vi "Update Fields Table for Spartan 5.0.vi"(8 "error in (no error)":errorcluster, 10 "spartan install dir":path, 11 "Connection Refnum":T1) -> (0 "error out":errorcluster, 2 "Map IndexName to FieldId":T2(array[cluster]), 3 "dup Connection Refnum":T1)   [LabVIEW 2011]
uses:
  SI.LIB/ODBC/SQL Controls/Connection Refnum.ctl
  Field Order By.ctl
  Field DataTypes.ctl
  Field Record.ctl
  Field NextItem.ctl
panel:
  out "array":string[](array[string])
  out "Array":errorcluster[](array[cluster])
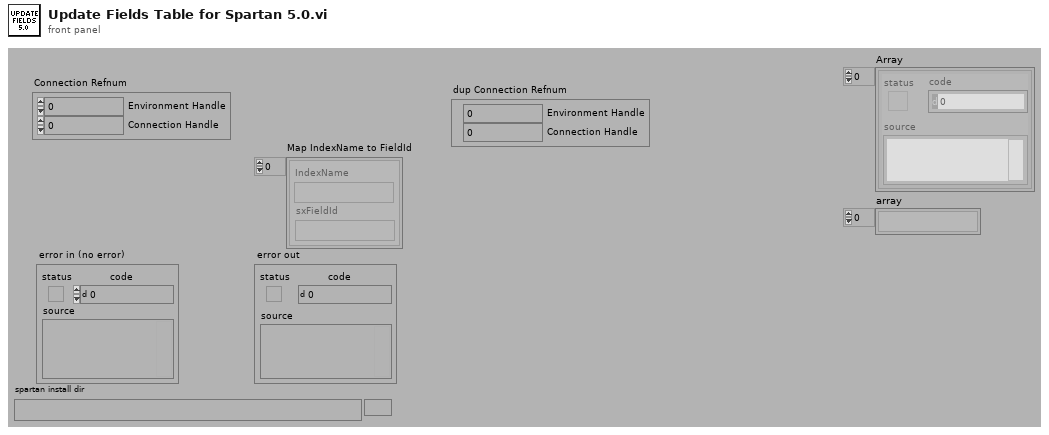
[diagram p1: front panel]
types:
  T1 = typedef "Connection Refnum.ctl" = cluster{"Environment Handle":i32, "Connection Handle":i32}
  T2 = cluster{"IndexName":string, "sxFieldId":string}[]
  T3 = typedef "Field Record.ctl" = cluster{"ixField":i32, "iSequenceOrder":i32, "sxFieldId":string, "sxSequenceId":string, "sDisplayName":string, "sValue":string, "sUnits":string, "nDataType":T4, "nNextItem":T5, "fSystem":bool, "fSystemValue":bool, "fRequired":bool, "fSetAtTest":bool, "fTestField":bool, "fDeleted":bool, "fIndexed":bool, "fFreeList":bool}
  T4 = typedef "Field DataTypes.ctl" = enum32{"text", "numeric", "list", "timestamp", "boolean"}
  T5 = typedef "Field NextItem.ctl" = enum32{"Reset", "Retain", "Auto-Increment"}
  T6 = enum16{"tdm_file", "tdm_channelgroup", "tdm_channel"}
  T7 = typedef "Field Order By.ctl" = enum32{"sxSequenceId", "sxFieldId", "sDisplayName", "sValue", "fSetAtTest", "fRequired", "nNextItem"}
  T8 = typedef "Statement Refnum.ctl" = cluster{"Statement Handle":i32, "Parameter Number":u16}
  T9 = typedef "DataFinder Indexed Property DataTypes.ctl" = enum32{"not optimized", "string", "double", "integer"}
  T10 = cluster{"DisplayName":string, "DataType":T9, "BuiltIn":bool}[]
  T11 = cluster{"DisplayName":string, "sxFieldId":string}
  T12 = cluster{"DisplayName":string, "sxFieldId":string}[]
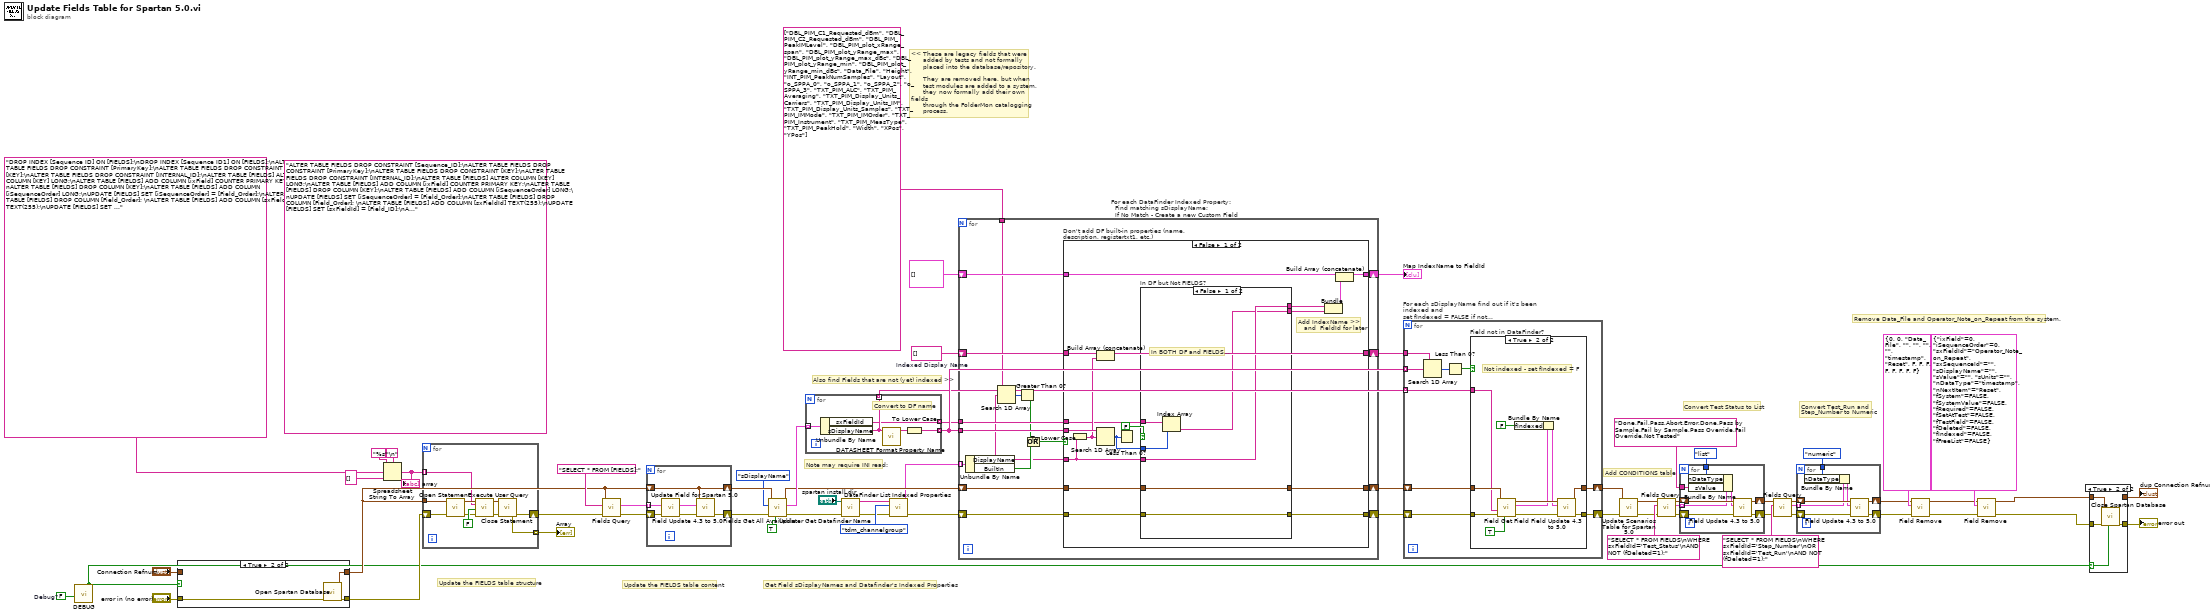
[diagram p0: block diagram]
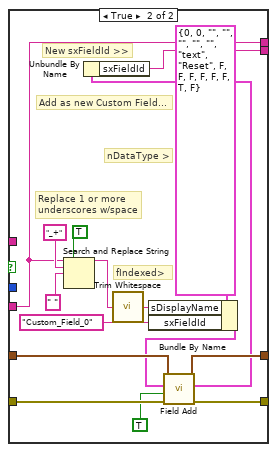
[diagram p5: hidden frame]
diagram:
  w7 = FALSE  # Debug?
  (unwired) "ALTER TABLE FIELDS DROP CONSTRAINT [Sequence_ID];\nALTER TABLE FIELDS DROP CONSTRAINT [PrimaryKey];\nALTER TABLE FIELDS DROP CONSTRAINT [KEY];\nALTER TABLE FIELDS DROP CONSTRAINT [INTERNAL_ID];\nALTER TABLE [FIELDS] ALTER COLUMN [KEY] LONG;\nALTER TABLE [FIELDS] ADD COLUMN [ixField] COUNTER PRIMARY KEY;\nALTER TABLE [FIELDS] DROP COLUMN [KEY];\nALTER TABLE [FIELDS] ADD COLUMN [iSequenceOrder] LONG;\nUPDATE [FIELDS] SET [iSequenceOrder] = [Field_Order];\nALTER TABLE [FIELDS] DROP COLUMN [Field_Order]; \nALTER TABLE [FIELDS] ADD COLUMN [sxFieldId] TEXT(255);\nUPDATE [FIELDS] SET [sxFieldId] = [Field_ID];\nALTER TABLE [FIELDS] DROP COLUMN [Field_ID]; \nALTER TABLE [FIELDS] ADD COLUMN [sxSequenceId] TEXT(255);\nUPDATE [FIELDS] SET [sxSequenceId] = [Sequence_ID] WHERE Sequence_ID IS NOT NULL;\nALTER TABLE [FIELDS] ADD COLUMN [sDisplayName] TEXT(255);\nUPDATE [FIELDS] SET [sDisplayName] = [Display_Name];\nALTER TABLE [FIELDS] DROP COLUMN [Display_Name]; \nALTER TABLE [FIELDS] ADD COLUMN [sValue] TEXT(255);\nUPDATE [FIELDS] SET [sValue] = [Field_Value];\nALTER TABLE [FIELDS] DROP COLUMN [Field_Value];\nALTER TABLE [FIELDS] ADD COLUMN [sUnits] TEXT(255);\nALTER TABLE [FIELDS] ADD COLUMN [nDataType] LONG;\nALTER TABLE [FIELDS] ADD COLUMN [nNextItem] LONG;\nALTER TABLE [FIELDS] ADD COLUMN [fSystem] LONG;\nALTER TABLE [FIELDS] ADD COLUMN [fSystemValue] LONG;\nALTER TABLE [FIELDS] ADD COLUMN [fRequired] LONG;\nALTER TABLE [FIELDS] ADD COLUMN [fSetAtTest] LONG;\nALTER TABLE [FIELDS] ADD COLUMN [fTestField] LONG;\nALTER TABLE [FIELDS] ADD COLUMN [fDeleted] LONG;\nALTER TABLE [FIELDS] ADD COLUMN [fIndexed] LONG;\nALTER TABLE [FIELDS] ADD COLUMN [fFreeList] LONG;\nUPDATE [FIELDS] SET [sUnits] = [Properties];\nALTER TABLE [FIELDS] DROP COLUMN [Properties];\nALTER TABLE [FIELDS] DROP CONSTRAINT [SEQUENCESFIELDS];\nALTER TABLE [FIELDS] DROP COLUMN [Sequence_ID];" ("User Query")
  w53 = string[] []  # Indexed Display Name
  # "<< These are legacy fields that were\n      added by tests and not formally\n      placed into the database/repository.\n\n      They are removed here, but when\n      test modules are added to a system,\n      they now formally add their own fields\n      through the FolderMon catalogging\n      process."
  # "Note may require INI read:"
  # "Convert Test_Run and\nStep_Number to Numeric"
  # "Remove Data_File and Operator_Note_on_Repeat from the system."
  # "Convert Test Status to List"
  # "Also find Fields that are not (yet) indexed >>"
  # "Get Field sDisplayNames and Datafinder's Indexed Properties"
  # "Add CONDITIONS table"
  # "Update the FIELDS table content"
  # "Update the FIELDS table structure"
  n1 = call "DEBUG.vi"("Dev DEBUG? (f)"=w7) -> ("DEBUG?"=w6:bool)  [unwired: 1 in, 5 out]
  n2 = case shown="True" w6 {
    tunnel: "Connection Refnum" -> [w68 _]
    tunnel: "error in (no error)" -> [w67 w71]
    tunnel: [w67 w70] -> w11
    tunnel: [w68 w69] -> w13
    frame False {
    }
    frame True {
      n3 = call "Open Spartan Database.vi"("error in (no error)"=w71) -> ("error out"=w70:errorcluster, "Connection Refnum"=w69:T1)  [unwired: 2 in, 7 out]
    }
  }
  n4 = Spreadsheet String To Array(delimiter (Tab)="\n", format string="%s", spreadsheet string="DROP INDEX [Sequence ID] ON [FIELDS];\nDROP INDEX [Sequence ID1] ON [FIELDS];\nALTER TABLE FIELDS DROP CONSTRAINT [PrimaryKey];\nALTER TABLE FIELDS DROP CONSTRAINT [KEY];\nALTER TABLE FIELDS DROP CONSTRAINT [INTERNAL_ID];\nALTER TABLE [FIELDS] ALTER COLUMN [KEY] LONG;\nALTER TABLE [FIELDS] ADD COLUMN [ixField] COUNTER PRIMARY KEY;\nALTER TABLE [FIELDS] DROP COLUMN [KEY];\nALTER TABLE [FIELDS] ADD COLUMN [iSequenceOrder] LONG;\nUPDATE [FIELDS] SET [iSequenceOrder] = [Field_Order];\nALTER TABLE [FIELDS] DROP COLUMN [Field_Order]; \nALTER TABLE [FIELDS] ADD COLUMN [sxFieldId] TEXT(255);\nUPDATE [FIELDS] SET [sxFieldId] = [Field_ID];\nALTER TABLE [FIELDS] DROP COLUMN [Field_ID]; \nALTER TABLE [FIELDS] ADD COLUMN [sxSequenceId] TEXT(255);\nUPDATE [FIELDS] SET [sxSequenceId] = [Sequence_ID] WHERE Sequence_ID IS NOT NULL;\nALTER TABLE [FIELDS] ADD COLUMN [sDisplayName] TEXT(255);\nUPDATE [FIELDS] SET [sDisplayName] = [Display_Name];\nALTER TABLE [FIELDS] DROP COLUMN [Display_Name]; \nALTER TABLE [FIELDS] ADD COLUMN [sValue] TEXT(255);\nUPDATE [FIELDS] SET [sValue] = [Field_Value];\nALTER TABLE [FIELDS] DROP COLUMN [Field_Value];\nALTER TABLE [FIELDS] ADD COLUMN [sUnits] TEXT(255);\nALTER TABLE [FIELDS] ADD COLUMN [nDataType] LONG;\nALTER TABLE [FIELDS] ADD COLUMN [nNextItem] LONG;\nALTER TABLE [FIELDS] ADD COLUMN [fSystem] LONG;\nALTER TABLE [FIELDS] ADD COLUMN [fSystemValue] LONG;\nALTER TABLE [FIELDS] ADD COLUMN [fRequired] LONG;\nALTER TABLE [FIELDS] ADD COLUMN [fSetAtTest] LONG;\nALTER TABLE [FIELDS] ADD COLUMN [fTestField] LONG;\nALTER TABLE [FIELDS] ADD COLUMN [fDeleted] LONG;\nALTER TABLE [FIELDS] ADD COLUMN [fIndexed] LONG;\nALTER TABLE [FIELDS] ADD COLUMN [fFreeList] LONG;\nUPDATE [FIELDS] SET [sUnits] = [Properties];\nALTER TABLE [FIELDS] DROP COLUMN [Properties];\nALTER TABLE [FIELDS] DROP CONSTRAINT [SEQUENCESFIELDS];\nALTER TABLE [FIELDS] DROP COLUMN [Sequence_ID];" ("User Query"), array type (2D Dbl)=string[] []) -> (array=w65:string[])
  "array" <- w65
  n5 = for {
    tunnel: w13 -> [w77]
    tunnel: w65 -> [w73] mode=indexing
    tunnel: [w72] -> w5 mode=indexing
    shift-right: [w72] -> w33
    shift-left: w11 -> [w74]
    n6 = call "Open Statement.vi"("error in (no error)"=w74, "Connection Refnum"=w77) -> ("error out"=w79:errorcluster, "Statement Refnum"=w78:T8)  [unwired: 4 out]
    n7 = call "Execute User Query.vi"("error in (no error)"=w79, "Return Data? (f)"=FALSE, "User Query"=w73, "Statement Refnum"=w78) -> ("error out"=w75:errorcluster, "Statement Refnum"=w76:T8)  [unwired: 2 out]
    n8 = call "Close Statement.vi"("error in (no error)"=w75, "Statement Refnum"=w76) -> ("error out"=w72:errorcluster)  [unwired: 5 out]
  }
  "Array" <- w5
  n9 = call "Fields Query.vi"("error in (no error)"=w33, "Query"="SELECT * FROM [FIELDS];", "Connection Refnum"=w13) -> ("error out"=w61:errorcluster, "Fields"=w60:T3[])  [unwired: 1 in, 6 out]
  n10 = for {
    shift-right: [w86] -> w32
    shift-left: w61 -> [w83]
    shift-right: [w85] -> w59
    shift-left: w13 -> [w85]
    tunnel: w60 -> [w84] mode=indexing
    n11 = call "Update Field for Spartan 5.0.vi"("error in (no error)"=w83, "Old Field Record"=w84) -> ("error out"=w82:errorcluster, "New Field Record"=w81:T3)  [unwired: 8 out]
    n12 = call "Field Update 4.3 to 5.0.vi"("error in (no error)"=w82, "Field Record"=w81, "Connection Refnum"=w85) -> ("error out"=w86:errorcluster)  [unwired: 8 out]
  }
  n13 = call "Fields Get All Available.vi"("Combine All? (f)"=TRUE, "error in (no error)"=w32, "Sort by (sxSequenceId)"=Field_Order_By."sDisplayName", "Connection Refnum"=w59) -> ("error out"=w28:errorcluster, "System or ALL Combined Fields"=w55:T3[], "Connection Refnum"=w54:T1)  [unwired: 1 in, 4 out]
  n14 = for {
    tunnel: w55 -> [w91] mode=indexing
    tunnel: [w89] -> w49 mode=indexing
    tunnel: [w88] -> w48 mode=indexing
    tunnel: [w87] -> w46 mode=indexing
    # "Convert to DF name"
    n15 = Unbundle By Name(w91) -> ("sxFieldId"=w87:string, "sDisplayName"=w88:string)
    n16 = call "DATASHEET Format Property Name.vi"("String with \\r or \\n"=w88) -> ("String without \\r or \\n"=w90:string)  [unwired: 4 out]
    n17 = To Lower Case(string=w90) -> (all lower case string=w89:string)
  }
  n18 = call "Updater Get Datafinder Name.vi"("error in (no error)"=w28, "spartan install dir"="spartan install dir") -> ("error out"=w4:errorcluster, "datafinder name"=w3:string)  [unwired: 8 out]
  n19 = call "DataFinder List Indexed Properties.vi"("error in (no error)"=w4, "Type (tdm_file)"=T6."tdm_channelgroup", "DataFinder (\"My DataFinder\")"=w3) -> ("error out"=w29:errorcluster, "Indexed Properties"=w44:T10)  [unwired: 7 out]
  n20 = for "For each DataFinder Indexed Property:\n  Find matching sDisplayName;\n  If No Match - Create a new Custom Field" {
    shift-right: [w105] -> w30
    shift-left: w29 -> [w106]
    shift-right: [w107] -> w51
    shift-left: w54 -> [w108]
    tunnel: w49 -> [w104]
    shift-right: [w102] -> w52
    shift-left: w53 -> [w103]
    shift-right: [w100] -> w45
    shift-left: T2 [] ("IndexName to FieldId") -> [w101]
    tunnel: w46 -> [w99]
    tunnel: w44 -> [w98] mode=indexing
    tunnel: string[] ["DBL_PIM_C1_Requested_dBm", "DBL_PIM_C2_Requested_dBm", "DBL_PIM_PeakIMLevel", "DBL_PIM_plot_xRange_span", "DBL_PIM_plot_yRange_max", "DBL_PIM_plot_yRange_max_dBc", "DBL_PIM_plot_yRange_min", "DBL_PIM_plot_yRange_min_dBc", "Data_File", "Height", "INT_PIM_PeakNumSamples", "Layout", "o_SPPA_0", "o_SPPA_1", "o_SPPA_2", "o_SPPA_3", "TXT_PIM_ALC", "TXT_PIM_Averaging", "TXT_PIM_Display_Units_Carriers", "TXT_PIM_Display_Units_IM", "TXT_PIM_Display_Units_Samples", "TXT_PIM_IMMode", "TXT_PIM_IMOrder", "TXT_PIM_Instrument", "TXT_PIM_MeasType", "TXT_PIM_PeakHold", "Width", "XPos", "YPos"] ("Array") -> [w92]
    n21 = Unbundle By Name(w98) -> ("DisplayName"=w93:string, "BuiltIn"=w95:bool)
    n22 = Search 1D Array(1D array=w92, element=w93) -> (index of element=w97:i32)  [unwired: 1 out]
    n23 = Greater Than 0?(x=w97) -> (x > 0?=w96:bool)
    n24 = Or(x=w96, y=w95) -> (x .or. y?=w94:bool)
    n25 = case "Don't add DF built-in properties (name, description, registertxt1, etc.)" shown="False" w94 {
      tunnel: w108 -> [w124 w151]
      tunnel: [w123 w151] -> w107
      tunnel: w106 -> [w122 w150]
      tunnel: [w121 w150] -> w105
      tunnel: w93 -> [w120 _]
      tunnel: w104 -> [w125 _]
      tunnel: w103 -> [w119 w149]
      tunnel: [w117 w149] -> w102
      tunnel: w101 -> [w114 w148]
      tunnel: [w113 w148] -> w100
      tunnel: w99 -> [w116 _]
      frame False {
        # "Add IndexName >>\n   and  FieldId for later"
        n26 = To Lower Case(string=w120) -> (all lower case string=w118:string)
        n27 = Build Array (concatenate)(w119, w118) -> (w117:string[])
        n28 = Search 1D Array(1D array=w125, element=w118) -> (index of element=w115:i32)  [unwired: 1 out]
        n29 = Less Than 0?(x=w115) -> ()  [unwired: 1 out]
        n30 = case "In DF but Not FIELDS?" shown="False" FALSE {
          tunnel: w124 -> [w131 w145]
          tunnel: [w131 w144] -> w123
          tunnel: w122 -> [w130 w147]
          tunnel: [w130 w146] -> w121
          tunnel: w120 -> [w127 w134]
          tunnel: w116 -> [w129 _]
          tunnel: w115 -> [w128 _]
          tunnel: [w127 w134] -> w112
          tunnel: [w126 w132] -> w111
          frame False {
            # "In BOTH DF and FIELDS..."
            n31 = Index Array(array=w129, index=w128) -> (element=w126:string)
          }
          frame True {
            # "New sxFieldId >>"
            # "nDataType >"
            # "fIndexed>"
            # "Replace 1 or more\nunderscores w/space"
            # "Add as new Custom Field..."
            n32 = Search and Replace String(replace all?=TRUE, input string=w134, search string="_+" ("sxFieldId"), replace string=" " ("sxFieldId")) -> (result string=w139:string)  [unwired: 1 in, 6 out]
            n33 = call <vilib>:"Trim Whitespace.vi"("string"=w139) -> ("trimmed string"=w135:string)  [unwired: 1 in]
            n34 = Bundle By Name(cluster=T3 {"ixField"=0, "iSequenceOrder"=0, "sxFieldId"="", "sxSequenceId"="", "sDisplayName"="", "sValue"="", "sUnits"="", "nDataType"=enum."text", "nNextItem"=enum."Reset", "fSystem"=FALSE, "fSystemValue"=FALSE, "fRequired"=FALSE, "fSetAtTest"=FALSE, "fTestField"=FALSE, "fDeleted"=FALSE, "fIndexed"=TRUE, "fFreeList"=FALSE} ("Field Record"), "sDisplayName"=w135, "sxFieldId"="Custom_Field_0") -> (w140:T3)
            n35 = call "Field Add.vi"("error in (no error)"=w147, "Force Unique? (f)"=TRUE, "Field Record"=w140, "Connection Refnum"=w145) -> ("error out"=w146:errorcluster, "New Field"=w133:T3, "Connection Refnum"=w144:T1)  [unwired: 5 out]
            n36 = Unbundle By Name(w133) -> ("sxFieldId"=w132:string)
          }
        }
        n37 = Bundle("DisplayName"=w112, "sxFieldId"=w111) -> (w110:T11)  [unwired: 1 out]
        n38 = Build Array (concatenate)(w114, w110) -> (w113:T12)
      }
      frame True {
      }
    }
  }
  "Map IndexName to FieldId" <- w45
  n39 = for "For each sDisplayName find out if it's been indexed and\nset fIndexed = FALSE if not..." {
    shift-right: [w153] -> w50
    shift-left: w30 -> [w155]
    tunnel: w52 -> [w160]
    shift-right: [w154] -> w36
    shift-left: w51 -> [w156]
    tunnel: w49 -> [w157] mode=indexing
    tunnel: w48 -> [w152] mode=indexing
    n40 = Search 1D Array(1D array=w160, element=w157) -> (index of element=w159:i32)  [unwired: 1 out]
    n41 = Less Than 0?(x=w159) -> (x < 0?=w158:bool)
    n42 = case "Field not in DataFinder?" shown="True" w158 {
      tunnel: w156 -> [w162 w168]
      tunnel: w155 -> [w161 w171]
      tunnel: [w162 w172] -> w154
      tunnel: [w161 w173] -> w153
      tunnel: w152 -> [_ w166]
      frame False {
        # "fIndexed already set..."
      }
      frame True {
        # "Not indexed - set fIndexed = F"
        n43 = call "Field Get Field.vi"("by sDisplayName? (f, by sFieldId)"=TRUE, "error in (no error)"=w171, "sFieldId or sDisplayName (\"\")"=w166, "Connection Refnum"=w168) -> ("error out"=w170:errorcluster, "Field"=w165:T3, "Connection Refnum"=w169:T1)  [unwired: 1 in, 4 out]
        n44 = Bundle By Name(cluster=w165, "fIndexed"=FALSE) -> (w163:T3)
        n45 = call "Field Update 4.3 to 5.0.vi"("error in (no error)"=w170, "Field Record"=w163, "Connection Refnum"=w169) -> ("error out"=w173:errorcluster, "Connection Refnum"=w172:T1)  [unwired: 7 out]
      }
    }
  }
  n46 = call "Update Scenarios Table for Spartan 5.0.vi"("error in (no error)"=w50, "Connection Refnum"=w36) -> ("error out"=w31:errorcluster, "Connection Refnum"=w35:T1)  [unwired: 8 out]
  n47 = call "Fields Query.vi"("error in (no error)"=w31, "Query"="SELECT * FROM FIELDS\nWHERE sxFieldId='Test_Status'\nAND NOT (fDeleted=1);" ("sFieldId or sDisplayName (\"\")"), "Connection Refnum"=w35) -> ("error out"=w41:errorcluster, "Fields"=w38:T3[], "Connection Refnum"=w42:T1)  [unwired: 2 in, 4 out]
  n48 = for {
    tunnel: Field_DataTypes."list" ("nDataType") -> [w179]
    tunnel: "Done,Fail,Pass,Abort,Error,Done,Pass by Sample,Fail by Sample,Pass Override,Fail Override,Not Tested" ("sValue") -> [w178]
    tunnel: w38 -> [w175] mode=indexing
    shift-right: [w176] -> w21
    shift-left: w41 -> [w180]
    shift-right: [w174] -> w22
    shift-left: w42 -> [w181]
    n49 = Bundle By Name(cluster=w175, "nDataType"=w179, "sValue"=w178) -> (w177:T3)
    n50 = call "Field Update 4.3 to 5.0.vi"("error in (no error)"=w180, "Field Record"=w177, "Connection Refnum"=w181) -> ("error out"=w176:errorcluster, "Connection Refnum"=w174:T1)  [unwired: 7 out]
  }
  n51 = call "Fields Query.vi"("error in (no error)"=w21, "Query"="SELECT * FROM FIELDS\nWHERE sxFieldId='Step_Number'\nOR sxFieldId='Test_Run'\nAND NOT (fDeleted=1);" ("sFieldId or sDisplayName (\"\")"), "Connection Refnum"=w22) -> ("error out"=w24:errorcluster, "Fields"=w26:T3[], "Connection Refnum"=w23:T1)  [unwired: 2 in, 4 out]
  n52 = for {
    tunnel: Field_DataTypes."numeric" ("nDataType") -> [w186]
    tunnel: w26 -> [w183] mode=indexing
    shift-right: [w184] -> w19
    shift-left: w24 -> [w187]
    shift-right: [w182] -> w20
    shift-left: w23 -> [w188]
    n53 = Bundle By Name(cluster=w183, "nDataType"=w186) -> (w185:T3)
    n54 = call "Field Update 4.3 to 5.0.vi"("error in (no error)"=w187, "Field Record"=w185, "Connection Refnum"=w188) -> ("error out"=w184:errorcluster, "Connection Refnum"=w182:T1)  [unwired: 7 out]
  }
  n55 = call "Field Remove.vi"("error in (no error)"=w19, "Field Record"=T3 {"ixField"=0, "iSequenceOrder"=0, "sxFieldId"="Data_File", "sxSequenceId"="", "sDisplayName"="", "sValue"="", "sUnits"="", "nDataType"=enum."timestamp", "nNextItem"=enum."Reset", "fSystem"=FALSE, "fSystemValue"=FALSE, "fRequired"=FALSE, "fSetAtTest"=FALSE, "fTestField"=FALSE, "fDeleted"=FALSE, "fIndexed"=FALSE, "fFreeList"=FALSE}, "Connection Refnum"=w20) -> ("error out"=w17:errorcluster, "Connection Refnum"=w16:T1)  [unwired: 7 out]
  n56 = call "Field Remove.vi"("error in (no error)"=w17, "Field Record"=T3 {"ixField"=0, "iSequenceOrder"=0, "sxFieldId"="Operator_Note_on_Repeat", "sxSequenceId"="", "sDisplayName"="", "sValue"="", "sUnits"="", "nDataType"=enum."timestamp", "nNextItem"=enum."Reset", "fSystem"=FALSE, "fSystemValue"=FALSE, "fRequired"=FALSE, "fSetAtTest"=FALSE, "fTestField"=FALSE, "fDeleted"=FALSE, "fIndexed"=FALSE, "fFreeList"=FALSE}, "Connection Refnum"=w16) -> ("error out"=w9:errorcluster, "Connection Refnum"=w10:T1)  [unwired: 7 out]
  n57 = case shown="True" w6 {
    selector: w6 -> [_ w191]
    tunnel: w9 -> [w190 w194]
    tunnel: w10 -> [w189 w193]
    tunnel: [w190 w192] -> w8
    tunnel: [w189 _] -> w1
    frame False {
    }
    frame True {
      n58 = call "Close Spartan Database.vi"("Force Close? (f)"=w191, "error in (no error)"=w194, "Connection Refnum"=w193) -> ("error out"=w192:errorcluster)  [unwired: 2 in, 6 out]
    }
  }
  "error out" <- w8
  "dup Connection Refnum" <- w1
